vi "closeConnection.vi"(8 "error in (no error)":errorcluster, 11 "Arduino in":refnum<class "Arduino.lvclass">) -> (0 "error out":errorcluster, 3 "Arduino out":refnum<class "Arduino.lvclass">)   [LabVIEW 2020, in "Arduino.lvclass"]
uses:
  Arduino.lvclass
  Arduino.lvclass/Arduino.ctl
  Interfaces/Arduino Shield/Arduino Shield.lvclass
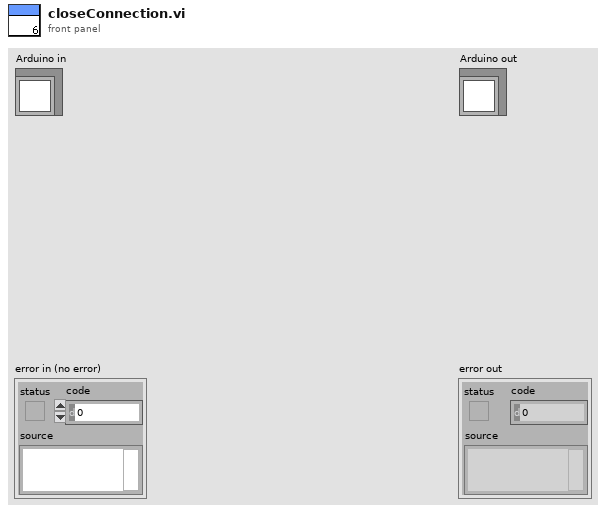
[diagram p1: front panel]
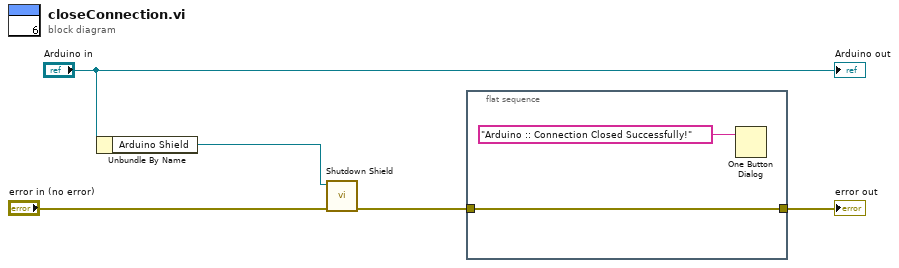
[diagram p0: block diagram]
diagram:
  n1 = Unbundle By Name("Arduino in") -> ("Arduino Shield"=w3:refnum<class "Arduino Shield.lvclass">)
  n2 = call-dynamic "Shutdown Shield.vi"("error in (no error)"="error in (no error)", "Arduino Shield in"=w3) -> ("error out"=w2:errorcluster)  [unwired: 8 in, 1 out]
  n3 = flat-sequence {
    tunnel: w2 -> [w6]
    tunnel: [w6] -> w1
    frame #0 {
      n4 = One Button Dialog(message="Arduino :: Connection Closed Successfully!") -> ()  [unwired: 1 in, 1 out]
    }
  }
  "error out" <- w1
  "Arduino out" <- "Arduino in"
